vi "Report Required Setting Missing Error.vi"(0 "Setting name":string, 11 "Error in (no error)":errorcluster) -> (15 "error out":errorcluster)   [LabVIEW 2023, in "RFCalAndFixtureCharact.Common.lvlib"]
uses:
  RFCalAndFixtureCharact.Common.lvlib
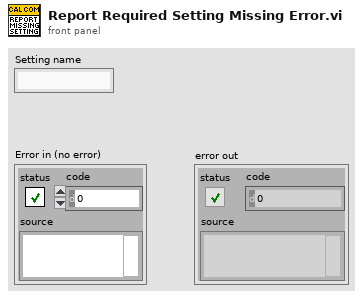
[diagram p1: front panel]
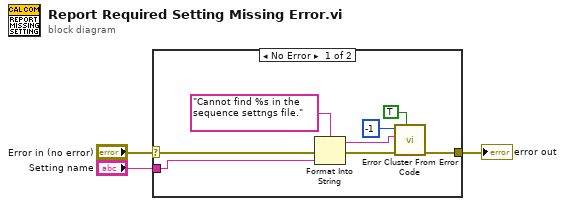
[diagram p0: block diagram]
diagram:
  n1 = case shown="No Error" "Error in (no error)" {
    selector: "Error in (no error)" -> [w9 w12]
    tunnel: [w10 w12] -> w2
    tunnel: "Setting name" -> [w6 _]
    frame No Error {
      n2 = Format Into String(format string="Cannot find %s in the sequence settngs file." ("error message (\"\")"), error in=w9, w6) -> (resulting string=w5:string, error out=w8:errorcluster)  [unwired: 1 in]
      n3 = call <vilib>:"Error Cluster From Error Code.vi"("show call chain? (False)"=TRUE, "error in (no error)"=w8, "error message (\"\")"=w5, "error code (0)"=-1) -> ("error out"=w10:errorcluster)  [unwired: 5 in]
    }
    frame Error {
    }
  }
  "error out" <- w2
